vi "niRFUtil WFM Remove Phase and Frequency Offset.vi"(0 "Waveform In":T2 {"y" format="%.2f"; "dx" format="%^.2e"; "x0" format="%^.2e"}, 5 "Reference Waveform In":T2 {"y" format="%.2f"; "dx" format="%^.2e"; "x0" format="%^.2e"}, 7 "Filter Phase Estimates":T1=enum."True", 9 "Filter Length (samples)":i32=20) -> (4 "Waveform Out":T2 {"y" format="%.2f"; "dx" format="%^.2e"; "x0" format="%^.2e"}, 6 "Reference Waveform Out":T2 {"y" format="%.2f"; "dx" format="%^.2e"; "x0" format="%^.2e"}, 13 "Frequency Offset (Hz)":sgl format="%^.2e", 14 "Phase Offset (deg)":sgl format="%.2f")   [LabVIEW 2015, in "niRFUtil.lvlib"]
doc: "(c) Copyright 2006, National Instruments, Inc. This VI may not be duplicated, sold, or distributed without written consent from National Instruments."
uses:
  niRFUtil.lvlib
  Includes/niRFUtil INC Complex Waveform.ctl
  Includes/niRFUtil INC Complex Array.ctl
  Includes/niRFUtil INC Filter Phase Estimates.ctl
  niRFUtil WFM Moving Average (complex array).vi
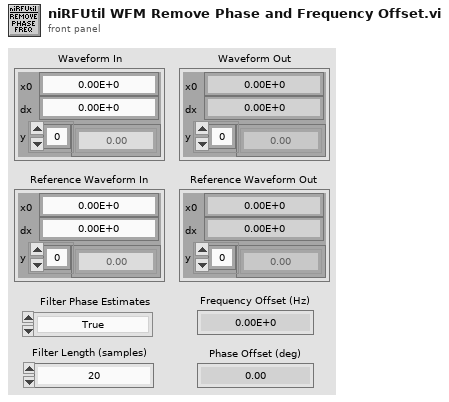
[diagram p1: front panel]
types:
  T1 = typedef "niRFUtil.lvlib/niRFUtil INC Filter Phase Estimates.ctl" = enum16{"False", "True"}
  T2 = typedef "niRFUtil.lvlib/niRFUtil INC Complex Waveform.ctl" = cluster{"x0":dbl, "dx":dbl, "y":T3}
  T3 = typedef "niRFUtil.lvlib/niRFUtil INC Complex Array.ctl" = csg[]
  T4 = typedef "niRFUtil.lvlib/niRFUtil INC Real Array.ctl" = sgl[]
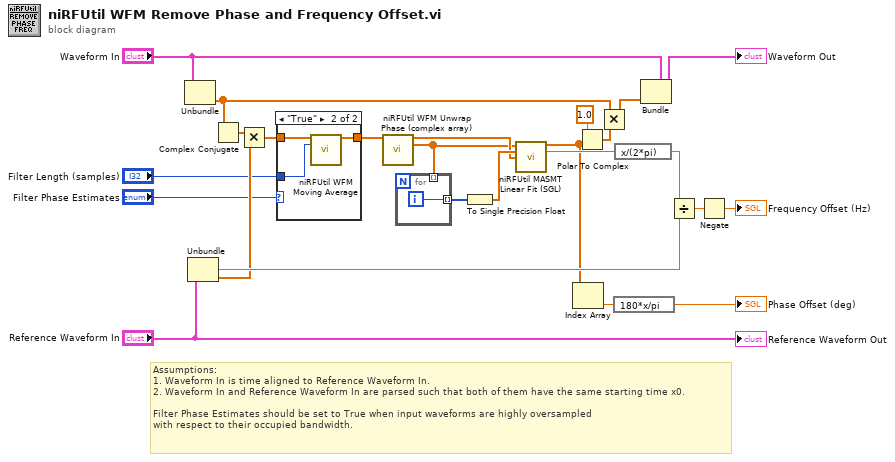
[diagram p0: block diagram]
diagram:
  # "Assumptions:\n1. Waveform In is time aligned to Reference Waveform In.\n2. Waveform In and Reference Waveform In are parsed such that both of them have the same starting time x0.\n\nFilter Phase Estimates should be set to True when input waveforms are highly oversampled\nwith respect to their occupied bandwidth."
  n1 = Unbundle("Waveform In") -> ("y"=w17:T3)  [unwired: 2 out]
  n2 = Unbundle("Reference Waveform In") -> ("dx"=w23:dbl, "y"=w7:T3)  [unwired: 1 out]
  n3 = Complex Conjugate(1:w17) -> (0:w25:T3)
  n4 = Multiply(x=w25, y=w7) -> (x*y=w6:T3)
  n5 = case shown="\"True\"" "Filter Phase Estimates" {
    tunnel: w6 -> [w26 w29]
    tunnel: [w26 w28] -> w5
    tunnel: "Filter Length (samples)" -> [_ w27]
    frame "False" {
    }
    frame "True" {
      n6 = call-poly "niRFUtil WFM Moving Average.vi"("Array In"=w29, "Averaging Window (samples)"=w27) -> ("Averaged Array Out"=w28:T3)  [unwired: 13 in]
    }
  }
  n7 = call "niRFUtil WFM Unwrap Phase (complex array).vi"("Complex Vectors"=w5) -> ("Magnitude"=w4:T4, "Unwrapped Phase (rad)"=w3:T4)  [unwired: 13 in]
  n8 = for {
    tunnel: [w30] -> w12 mode=indexing
    tunnel: w3 -> [_] mode=indexing
    i -> [w30]
  }
  n9 = To Single Precision Float(number=w12) -> (single precision float=w11:sgl[])
  n10 = call "niRFUtil MASMT Linear Fit (SGL).vi"("Y"=w3, "X"=w11, "Weight"=w4) -> ("Best Linear Fit"=w8:sgl[], "slope"=w20:sgl)  [unwired: 8 in, 3 out]
  n11 = Index Array(array=w8) -> (element=w10:sgl)  [unwired: 1 in]
  n12 = Polar To Complex(1:w8, 2:sgl 1.0) -> (0:w14:csg[])
  n13 = Multiply(x=w17, y=w14) -> (x*y=w16:T3)
  n14 = expression code="180*x/pi"(w10) -> (→"Phase Offset (deg)":sgl)
  n15 = expression code="x/(2*pi)"(w20) -> (w22:sgl)
  n16 = Bundle(cluster="Waveform In", "y"=w16) -> (→"Waveform Out":T2)  [unwired: 2 out]
  n17 = Divide(x=w22, y=w23) -> (x/y=w24:dbl)
  n18 = Negate(x=w24) -> (-x=→"Frequency Offset (Hz)":dbl)
  "Reference Waveform Out" <- "Reference Waveform In"
